vi "database_connection_write_DMMS_2.vi"(5 "ODBC data source name":string="amrc_monitoring", 6 "error in (no error)":errorcluster, 7 "G1?":u32, 8 "current time":timestamp, 9 "data 2":dbl[](array[numeric]), 10 "Machine Data":T1={"Zload"="", "Yload"="", "Xload"="", "path_position"="", "Fovr"="", "SspeedOvr"="", "Program Name"="", "Program status"="", "Block of code being executed"="", "Line of code"="", "Machine availability"="", "Emergency status"="", "Controller mode"="", "Tool_id"="UNAVAILABLE"}, 11 "Machine type":string) -> (3 "error out":errorcluster)   [LabVIEW 2017]
uses:
  <vilib>/addons/database/Connection.llb/DB Tools Open Connec (Path).vi
  <vilib>/addons/database/Connection.llb/Conn Execute.vi
  <vilib>/addons/database/Recordset.llb/Rec Destroy - Connection.vi
  <vilib>/regexp/Match Regular Expression.xnode
  <vilib>/addons/database/NI_Database_API.lvlib
panel:
  out "data 3":dbl[](array[numeric])
  out "path_position":string
  out "x = y?":bool
  out "submatch 1":string
  out "after match 3":string
  out "empty? 2":bool
  out "after match 2":string
  out "resulting string 4":string
  out "Xload":string
  out "concatenated string 6":string
  out "resulting string 3":string
  out "concatenated string 2":string
  out "resulting string 2":string
  out "ODBC data source name 2":string="amrc_monitoring"
  out "resulting string":string
  out "size(s)":i32
  out "concatenated string 5":string
  out "concatenated string 3":string
  out "concatenated string":string
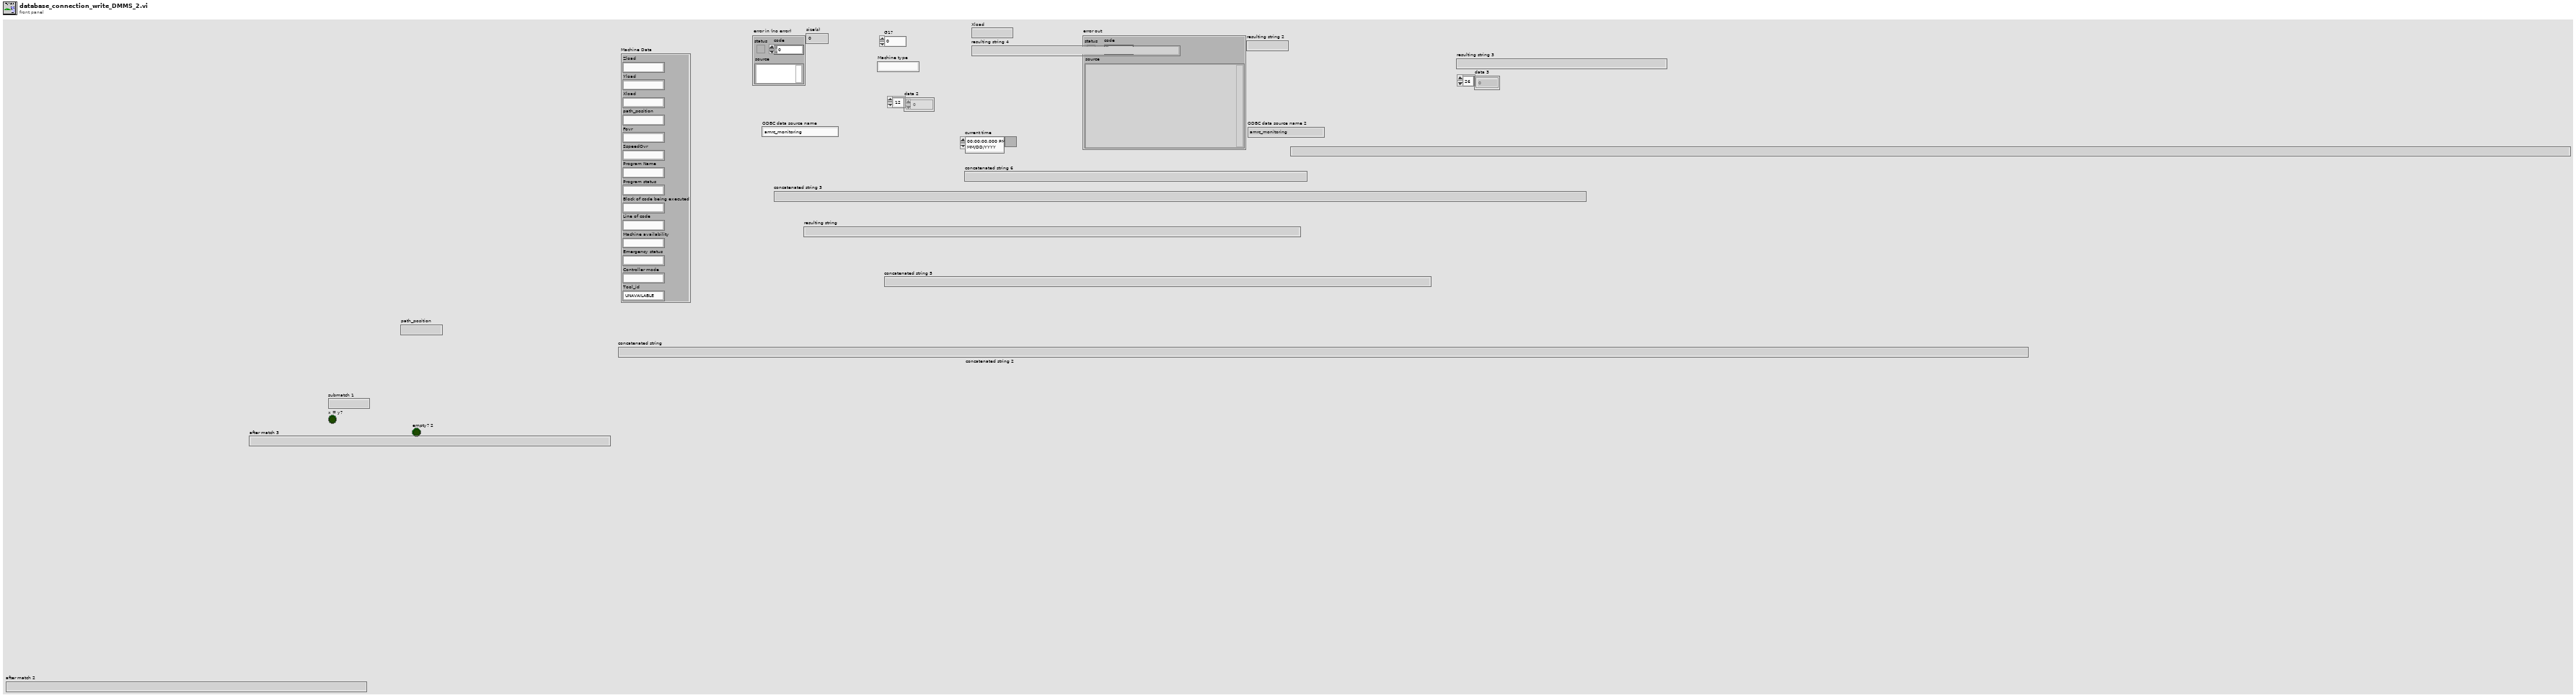
[diagram p1: front panel]
types:
  T1 = cluster{"Zload":string, "Yload":string, "Xload":string, "path_position":string, "Fovr":string, "SspeedOvr":string, "Program Name":string, "Program status":string, "Block of code being executed":string, "Line of code":string, "Machine availability":string, "Emergency status":string, "Controller mode":string, "Tool_id":string}
  T2 = typedef "NI_Database_API.lvlib/Conn ObjectReference.ctl" = refnum<k1>
  T3 = typedef "NI_Database_API.lvlib/Rec ObjectReference.ctl" = refnum<k1>
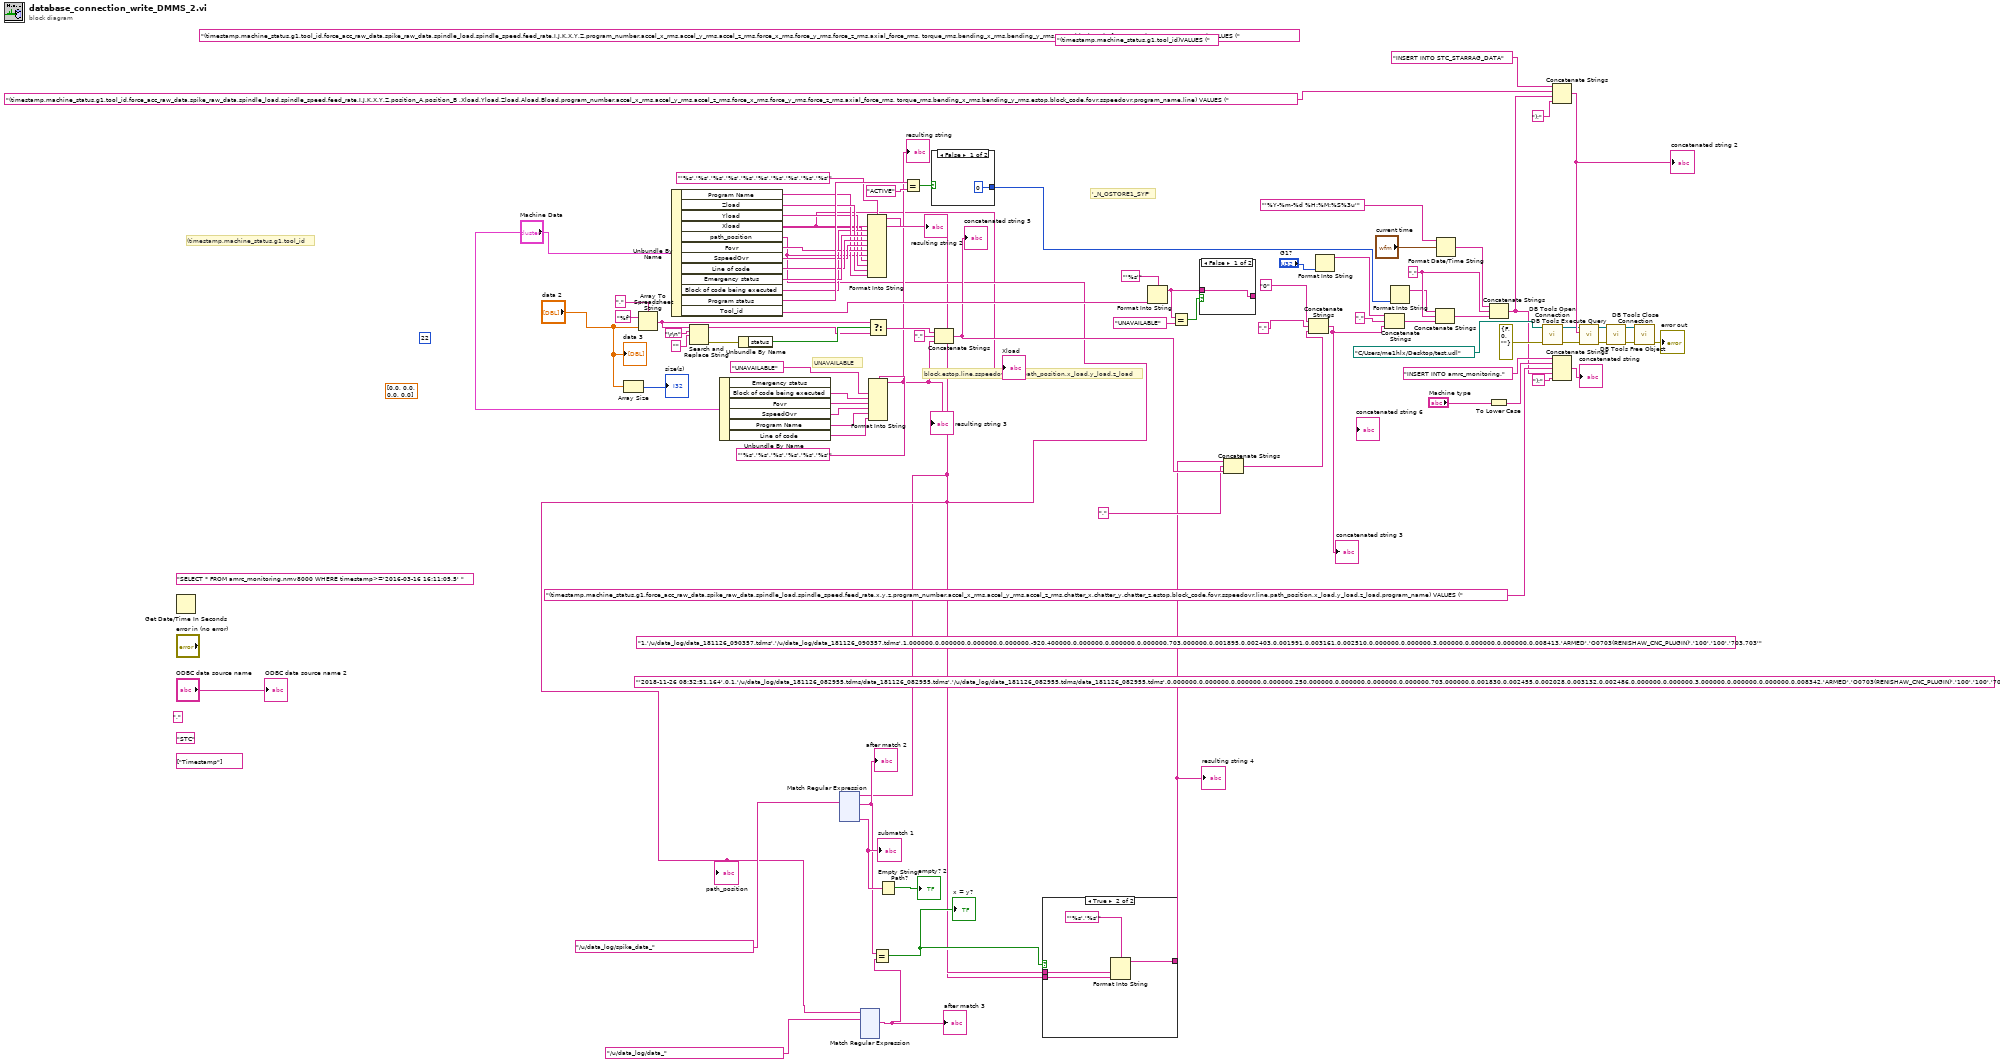
[diagram p0: block diagram]
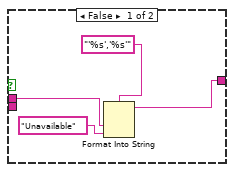
[diagram p2: hidden frame]
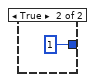
[diagram p4: hidden frame]
diagram:
  (unwired) "(timestamp,machine_status,g1,tool_id,force_acc_raw_data,spike_raw_data,spindle_load,spindle_speed,feed_rate,I,J,K,X,Y,Z,program_number,accel_x_rms,accel_y_rms,accel_z_rms,force_x_rms,force_y_rms,force_z_rms,axial_force_rms, torque_rms,bending_x_rms,bending_y_rms,estop,block_code,fovr,sspeedovr,program_name) VALUES (" ("string")
  (unwired) "(timestamp,machine_status,g1,tool_id)VALUES (" ("string")
  (unwired) dbl[] [0.0, 0.0, 0.0, 0.0]
  (unwired) "1,'/u/data_log/data_181126_090357.tdms','/u/data_log/data_181126_090357.tdms',1.000000,0.000000,0.000000,0.000000,-920.400000,0.000000,0.000000,0.000000,703.000000,0.001895,0.002403,0.001991,0.003161,0.002510,0.000000,0.000000,3.000000,0.000000,0.000000,0.008413,'ARMED','O0703(RENISHAW_CNC_PLUGIN)','100','100','703.703'" ("concatenated string 4")
  (unwired) "'2018-11-26 08:32:51.164',0,1,'/u/data_log/data_181126_082955.tdms/data_181126_082955.tdms','/u/data_log/data_181126_082955.tdms/data_181126_082955.tdms',0.000000,0.000000,0.000000,0.000000,250.000000,0.000000,0.000000,0.000000,703.000000,0.001830,0.002455,0.002028,0.003132,0.002486,0.000000,0.000000,3.000000,0.000000,0.000000,0.008342,'ARMED','O0703(RENISHAW_CNC_PLUGIN)','100','100','703.703'" ("concatenated string 2")
  (unwired) 22
  (unwired) "," ("string")
  (unwired) string[] ["Timestamp"]
  (unwired) "STC"
  w46 = "," ("string")
  (unwired) "SELECT * FROM amrc_monitoring.nmv8000 WHERE timestamp>='2016-03-16 16:11:05.5' " ("SQL query")
  # "(timestamp,machine_status,g1,tool_id"
  # "'_N_OSTORE1_SYF'"
  # "UNAVAILABLE"
  # "block,estop,line,sspeedovr,fovr,path_position,x_load,y_load,z_load"
  n1 = Get Date/Time In Seconds() -> ()  [unwired: 1 out]
  n2 = Array Size(array="data 2") -> (size(s)=→"size(s)":i32)
  n3 = Array To Spreadsheet String(delimiter (Tab)=",", array="data 2", 3:"%f" ("format string")) -> (spreadsheet string=w72:string)
  n4 = Unbundle By Name("Machine Data") -> ("Program Name"=w59:string, "Zload"=w63:string, "Yload"=w24:string, "Xload"=w3:string, "path_position"=w4:string, "Fovr"=w64:string, "SspeedOvr"=w65:string, "Line of code"=w66:string, "Emergency status"=w67:string, "Block of code being executed"=w57:string, "Program status"=w85:string, "Tool_id"=w51:string)
  "Xload" <- w3
  "path_position" <- w4
  n5 = Search and Replace String(input string=w72, search string="\r\n", replace string="" ("replace string (\"\")")) -> (result string=w73:string, error out=w75:errorcluster)  [unwired: 5 in, 2 out]
  n6 = Unbundle By Name("Machine Data") -> ("Block of code being executed"=w31:string, "Fovr"=w30:string, "SspeedOvr"=w29:string, "Program Name"=w28:string, "Line of code"=w1:string)  [unwired: 1 out]
  n7 = Unbundle By Name(w75) -> ("status"=w74:bool)
  n8 = xnode "Match Regular Expression"("input string"=w3, "regular expression"="/u/data_log/spike_data_") -> ("after match"=w7:string, "submatch 1"=w8:string)  [unwired: 4 in, 4 out]
  "after match 2" <- w7
  "submatch 1" <- w8
  n9 = xnode "Match Regular Expression"("input string"=w4, "regular expression"="/u/data_log/data_") -> ("after match"=w6:string)  [unwired: 4 in, 5 out]
  "after match 3" <- w6
  n10 = Format Into String(format string="'%s','%s','%s','%s','%s','%s','%s','%s','%s','%s'", w57, w67, w66, w65, w64, w4, w3, w24, w63, w59) -> (resulting string=→"resulting string 2":string)  [unwired: 2 in, 1 out]
  n11 = Select(t=w72, s=w74, f=w73) -> (s? t:f=w60:string)
  n12 = Format Into String(format string="'%s','%s','%s','%s','%s','%s'", "UNAVAILABLE" ("format string"), w31, w30, w29, w28, w1) -> (resulting string=w23:string)  [unwired: 2 in, 1 out]
  "resulting string" <- w23
  "resulting string 3" <- w23
  n13 = Equal?(x=w7, y=w6) -> (x = y?=w5:bool)
  "x = y?" <- w5
  n14 = Empty String/Path?(string/path=w8) -> (empty?=→"empty? 2":bool)
  n15 = Equal?(x=w85, y="ACTIVE") -> (x = y?=w83:bool)
  n16 = case shown="False" w83 {
    tunnel: [0 1] -> w19
    frame False {
    }
    frame True {
    }
  }
  n17 = Concatenate Strings(w60, "," ("string"), w23) -> (w15:string)
  "concatenated string 5" <- w15
  n18 = case shown="True" w5 {
    tunnel: w4 -> [w92 w94]
    tunnel: w3 -> [_ w97]
    tunnel: [w91 w95] -> w2
    frame False {
      n19 = Format Into String(format string="'%s','%s'", w92, "Unavailable" ("Tool_id")) -> (resulting string=w91:string)  [unwired: 2 in, 1 out]
    }
    frame True {
      n20 = Format Into String(format string="'%s','%s'", w94, w97) -> (resulting string=w95:string)  [unwired: 2 in, 1 out]
    }
  }
  "resulting string 4" <- w2
  n21 = Format Into String(format string="'%s'", w51) -> (resulting string=w50:string)  [unwired: 2 in, 1 out]
  n22 = Equal?(x=w50, y="UNAVAILABLE") -> (x = y?=w82:bool)
  n23 = case shown="False" w82 {
    tunnel: w50 -> [w98 w99]
    tunnel: [w98 w99] -> _
    frame False {
    }
    frame True {
    }
  }
  n24 = Concatenate Strings(w2, "," ("string"), w15) -> (w13:string)
  n25 = Concatenate Strings("0", "," ("string"), w13) -> (w20:string)
  "concatenated string 3" <- w20
  n26 = Format Into String("G1?") -> (resulting string=w44:string)  [unwired: 3 in, 1 out]
  n27 = Concatenate Strings(w44, "," ("string"), w20) -> (w22:string)
  n28 = Format Into String(w19) -> (resulting string=w45:string)  [unwired: 3 in, 1 out]
  n29 = Concatenate Strings(w45, w46, w22) -> (w78:string)
  n30 = Format Date/Time String(time format string (%c)="'%Y-%m-%d %H:%M:%S%3u'", seconds (now)="current time") -> (date/time string=w47:string)  [unwired: 1 in]
  n31 = To Lower Case(string="Machine type") -> (all lower case string=w69:string)
  n32 = Concatenate Strings(w47, w46, w78) -> (w21:string)
  n33 = call-poly <vilib>:"DB Tools Open Connection.vi"("error in (no error)"=errorcluster {"status"=FALSE, "code"=0, "source"=""}, "connection information"=path "C:/Users/me1hlx/Desktop/test.udl") -> ("error out"=w42:errorcluster, "connection reference"=w36:T2)  [unwired: 6 in]
  n34 = Concatenate Strings("INSERT INTO STC_STARRAG_DATA" ("string"), "(timestamp,machine_status,g1,tool_id,force_acc_raw_data,spike_raw_data,spindle_load,spindle_speed,feed_rate,I,J,K,X,Y,Z,position_A,position_B ,Xload,Yload,Zload,Aload,Bload,program_number,accel_x_rms,accel_y_rms,accel_z_rms,force_x_rms,force_y_rms,force_z_rms,axial_force_rms, torque_rms,bending_x_rms,bending_y_rms,estop,block_code,fovr,sspeedovr,program_name,line) VALUES (" ("string"), w21, ");" ("string")) -> (w43:string)
  "concatenated string 2" <- w43
  n35 = Concatenate Strings("INSERT INTO amrc_monitoring." ("string"), w69, "(timestamp,machine_status,g1,force_acc_raw_data,spike_raw_data,spindle_load,spindle_speed,feed_rate,x,y,z,program_number,accel_x_rms,accel_y_rms,accel_z_rms,chatter_x,chatter_y,chatter_z,estop,block_code,fovr,sspeedovr,line,path_position,x_load,y_load,z_load,program_name) VALUES (" ("string"), w21, ");" ("string")) -> (→"concatenated string":string)
  n36 = call-poly <vilib>:"DB Tools Execute Query.vi"("error in (no error)"=w42, "SQL query"=w43, "connection reference"=w36) -> ("error out"=w39:errorcluster, "recordset reference"=w40:T3)  [unwired: 5 in]
  n37 = call-poly <vilib>:"DB Tools Free Object.vi"("error in (no error)"=w39, "recordset reference"=w40) -> ("error out"=w37:errorcluster, "connection reference"=w38:T2)  [unwired: 8 in]
  n38 = call <vilib>:"DB Tools Close Connection.vi"("error in (no error)"=w37, "connection reference"=w38) -> ("error out"=→"error out":errorcluster)  [unwired: 5 in]
  "ODBC data source name 2" <- "ODBC data source name"
  "data 3" <- "data 2"
